vi "Program Oscillators.vi"(2 "Error In":errorcluster) -> (0 "Error Out":errorcluster)   [LabVIEW 2018]
uses:
  Type Defs/State Machine.ctl
  Type Defs/RT Command.ctl
  Type Defs/Global Action.ctl
  FGVs/Global Variables.vi
  <vilib>/Utility/config.llb/Read Key (U32).vi
  <vilib>/Utility/config.llb/Write Key (Double).vi
  <vilib>/Utility/config.llb/Write Key (Boolean).vi
  <vilib>/Utility/config.llb/NI_LVConfig.lvlib
panel:
  out "Register 0, 1, 6, 7":u32
  out "Frequncy Tuning Word":u32
  out "Register 7":u8 format="%x"
  out "Register 6":u8 format="%x"
  out "Register 5":u8 format="%x"
  out "Register 4":u8 format="%x"
  out "Register 3":u8 format="%x"
  out "Register 2":u8 format="%x"
  out "Register 1":u8 format="%x"
  out "Register 0":u8 format="%x"
  in  "Amplitude Scale Factor":dbl
  in  "Frequency Out":dbl
  in  "Reference Clock Multiplier":dbl
  in  "Reference Clock (Mhz)":dbl
  in  "DDS Select":u32(ring) items=["MP 1 - FREQ", "Q1 - FERQ", "Q2 - FREQ"]
  in  "Program Osc":bool
  in  "Current  Osc Settings":bool
  # "(160 + the Reference Clock Multipler value)"
  # "(193, the value to select single tone mode, \nDPD pin for shutdown, no SLEEP mode)"
  # "(the 1st 8 bits of the frequency tuning word)"
  # "(the 2nd 8 bits of the frequency tuning word)"
  # "(the 3rd 8 bits of the frequency tuning word)"
  # "(the last 8 bits of the frequency tuning word)"
  # "(5, the value to bypass the CIC filter)"
  # "(128 * the Amplitude Scale Factor)"
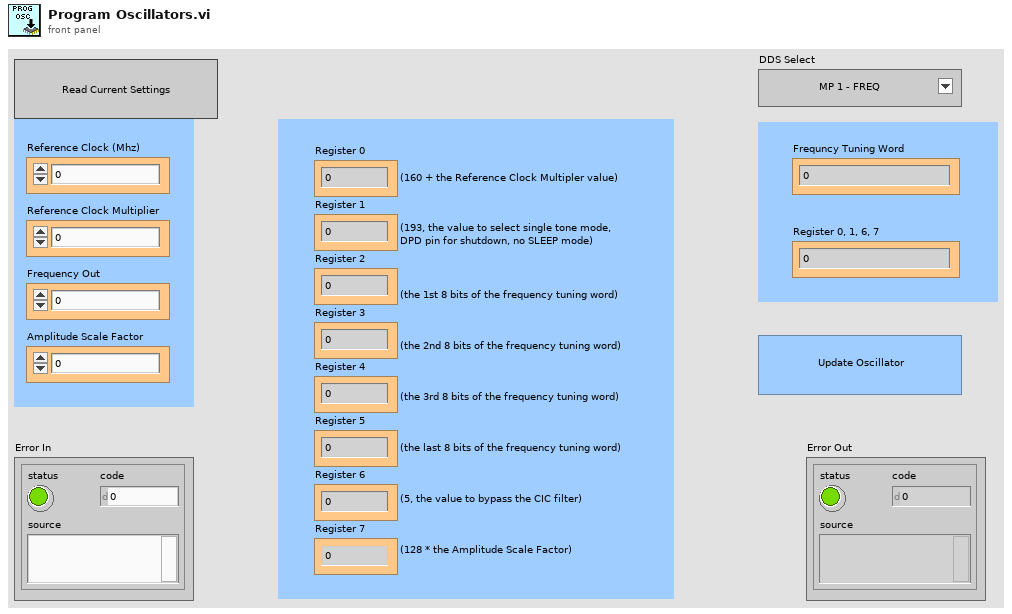
[diagram p1: front panel]
types:
  T1 = typedef "State Machine.ctl" = enum16{"Case 0", "Case 1", "Case 2", "Case 3", "Case 4", "Case 5", "Case 6", "Case 7", "Case 8", "Case 9", "Case 10", "Error", "Exit"}
  T2 = enum8{"Enabled", "Disabled", "Disabled and Grayed Out"}
  T3 = typedef "Global Action.ctl" = enum16{"Write", "Read"}
  T4 = typedef "RT Command.ctl" = enum16{"xml Start Run", "xml Start Actual Run", "xml Stop Run", "xml Runtime Update", "xml Get Status", "xml Get Table", "xml Set Table", "xml Get Configuration", "xml System Status", "xml Set LC Input Logic", "xml Get Data", "xml Get Info", "Start", "StartActualRun", "Stop", "Runtime Update", "Get Data", "Get Info", "Get Status", "Get Param", "Get Config", "Get Table", "Read ADC", "Set Oscillator", "Update Config", "Update Table", "Set All Pol", "Set Pol and DC", "Set Max Mass", "Toggle RP", "Toggle EL", "Set PIC", "Initialize Turbo", "Send Turbo Comm", "Close Turbo", "P1", "P2", "P3", "Send Serial", "Set LC Out", "Get LC In", "Read VAC", "Test Table", "Toggle Power", "Get Startup", "Set Startup", "Get ADC Table", "Set ADC Table", "Get Brief Status", "Get Detail Status", "Auxiliary Update", "Set CC Logics", "Set CC Input Logics", "Ignore Error", "invalid"}
  T5 = typedef "NI_LVConfig.lvlib/Config Data RefNum.ctl" = refnum<k1>
  T6 = typedef "Global Configrations.ctl" = cluster{"Model Name":enum16{"QSight 110", "QSight 120", "QSight 210", "QSight 220", "QSight 410", "QSight 420", "IONICS 3Q 110", "IONICS 3Q 120", "IONICS 3Q 210", "IONICS 3Q 220", "IONICS 3Q 310", "IONICS 3Q 320", "Simulation (Single Source)", "Simulation (Dual Source)"}, "RunType":u16, "Acquisition State":enum16{"Ready", "Busy", "Waiting"}, "InstrState":enum16{"Initializing", "Mass Spectrometer is Off", "Starting Up", "Turning Power Off", "Going to Standby", "Roughing Pump Ready", "Turning Turbo Off", "Turbo Startup", "Turbopump Ready", "Checking Vacuum", "Going to Ready", "Ready", "Running", "Source Standby", "Lost Communication", "Shutting Down", "Fault", "24V Standby", "Go to 24V Standby", "Turbopump Ready-Waiting"}, "Run Mode":enum16{"MRM (Q1/Q2)", "Q1 Scan", "Q1 SRM", "Q2 Scan", "Q2 SRM", "Product Scan", "Precursor Scan", "Neutral Loss", "Neutral Gain"}, "Configration":T7, "TCP ID":refnum<k5>, "DT":bool, "Dead Time (nS)":i32, "Single Source":bool, "ADC Tables":T9[]}
  T7 = typedef "Configration.ctl" = cluster{"Table":T8[], "Instrument":string[]}
  T8 = typedef "_RT Configuration 2.ctl" = cluster{"Name":string, "Ch#":u8, "Min":dbl, "Max":dbl, "Def+":dbl, "Def-":dbl, "Offset":dbl, "Slope":dbl, "Type":u8, "Description":string, "SettleT":dbl}
  T9 = typedef "ADC Table.ctl" = cluster{"Name":string, "Ch#":u8, "Min":dbl, "Max":dbl, "Def+":dbl, "Def-":dbl, "Offset":dbl, "Slope":dbl, "Type":u8, "Description":string, "SettleT":dbl}
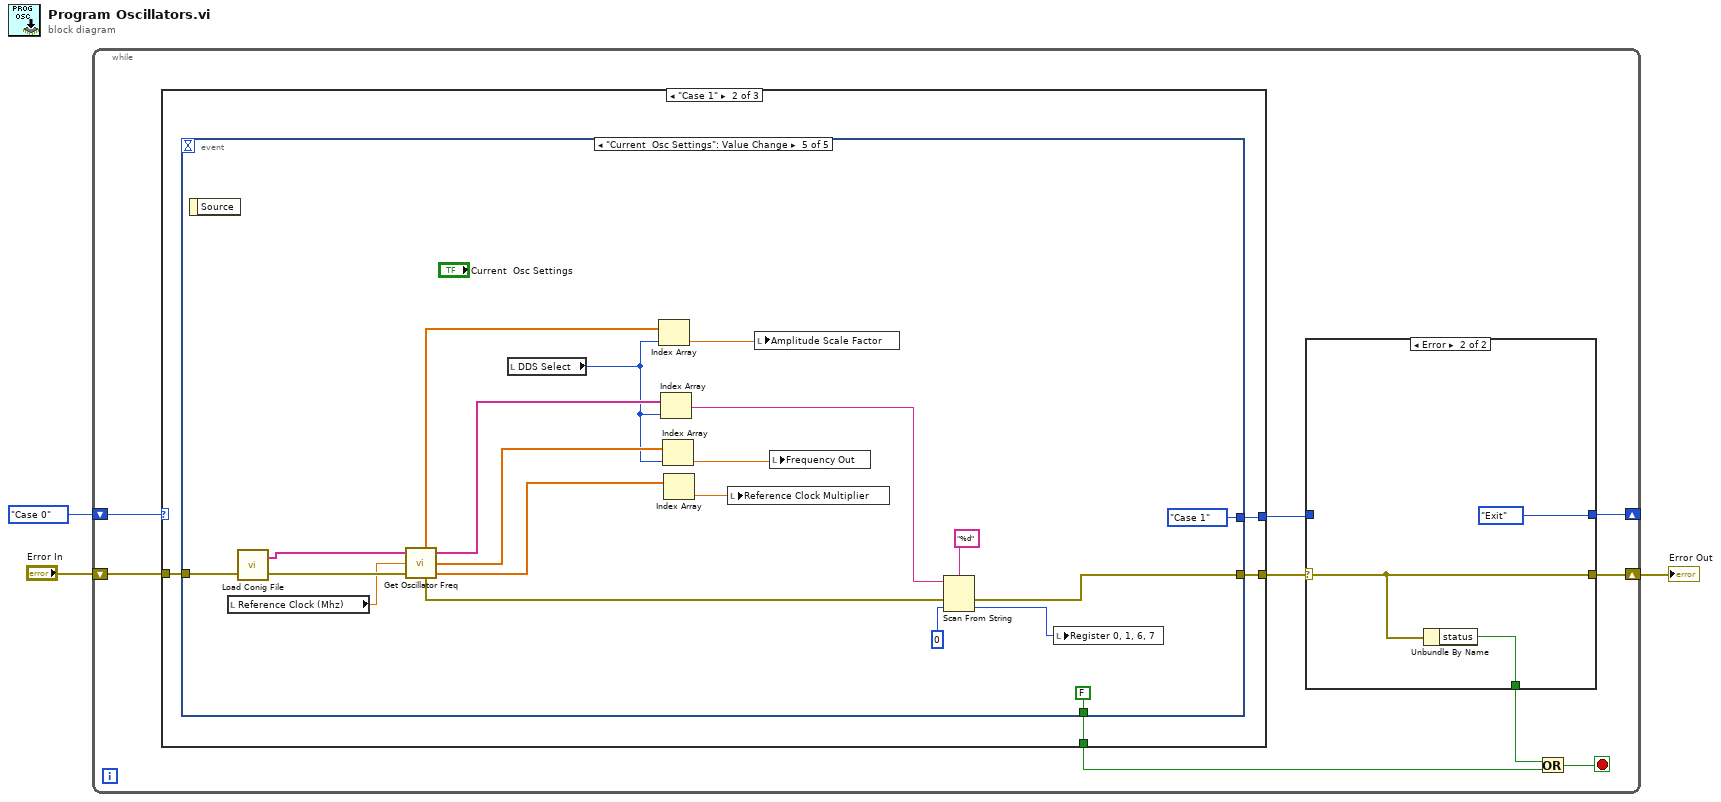
[diagram p0: block diagram]
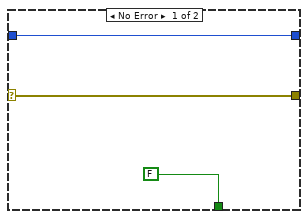
[diagram p2: hidden frame]
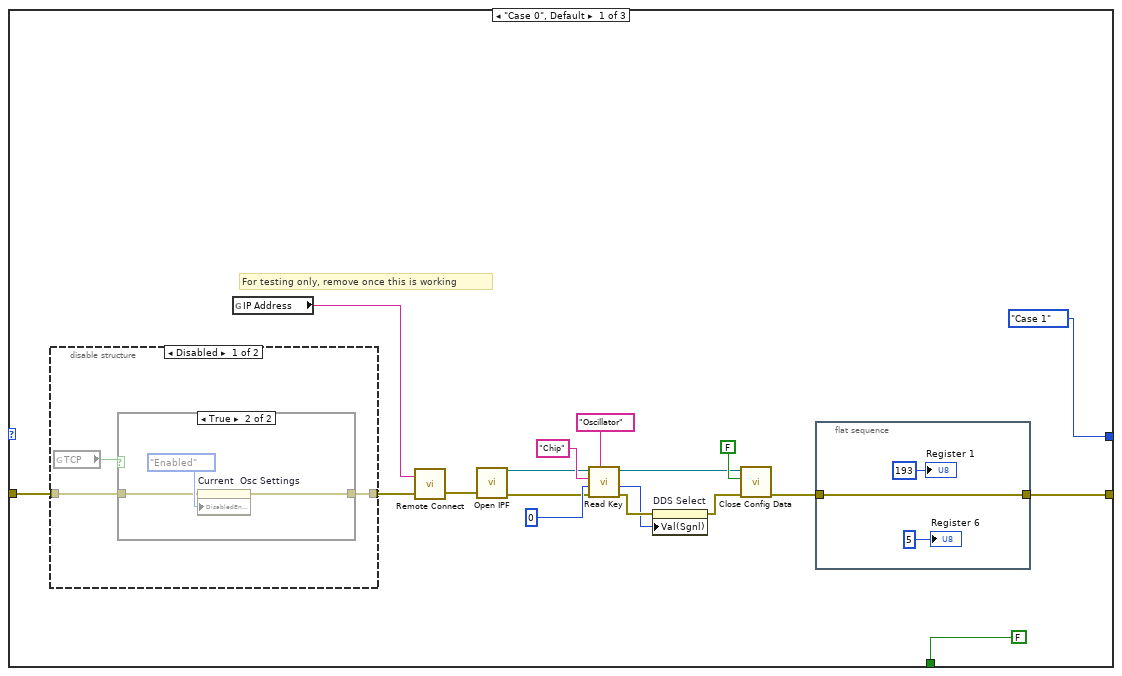
[diagram p3: hidden frame]
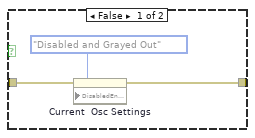
[diagram p4: hidden frame]
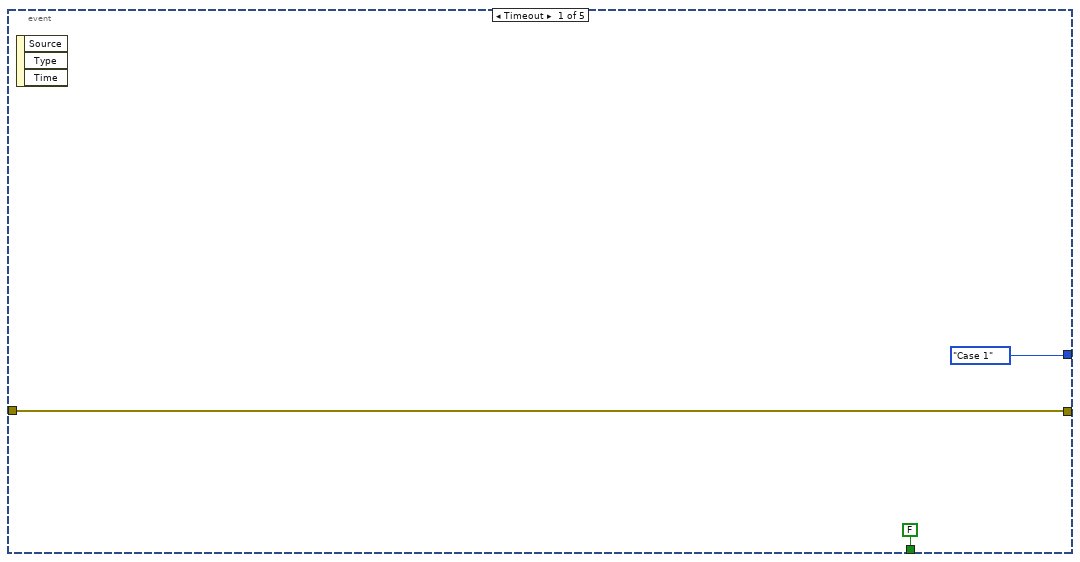
[diagram p6: hidden frame]
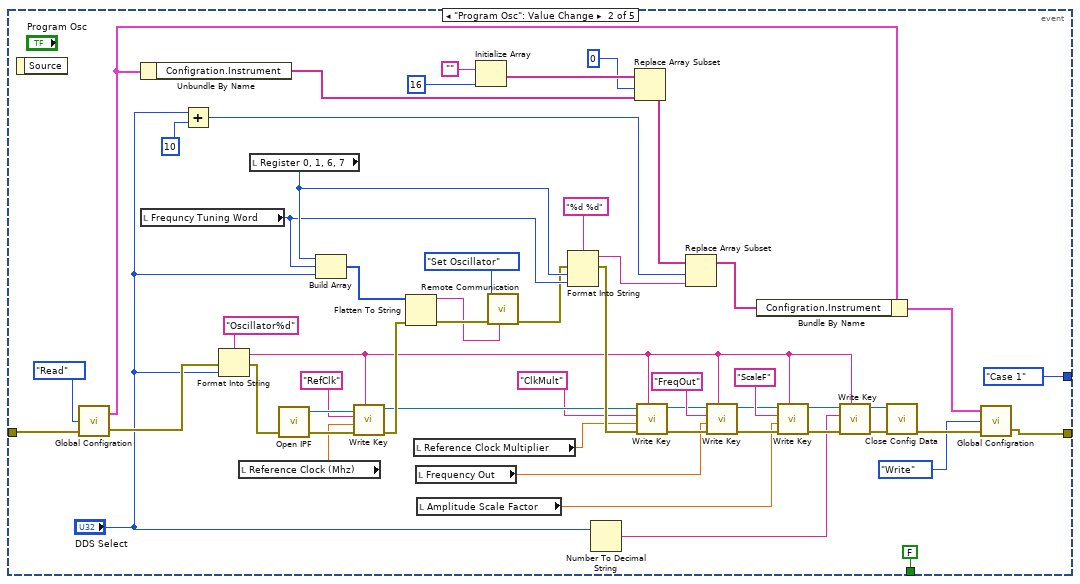
[diagram p7: hidden frame]
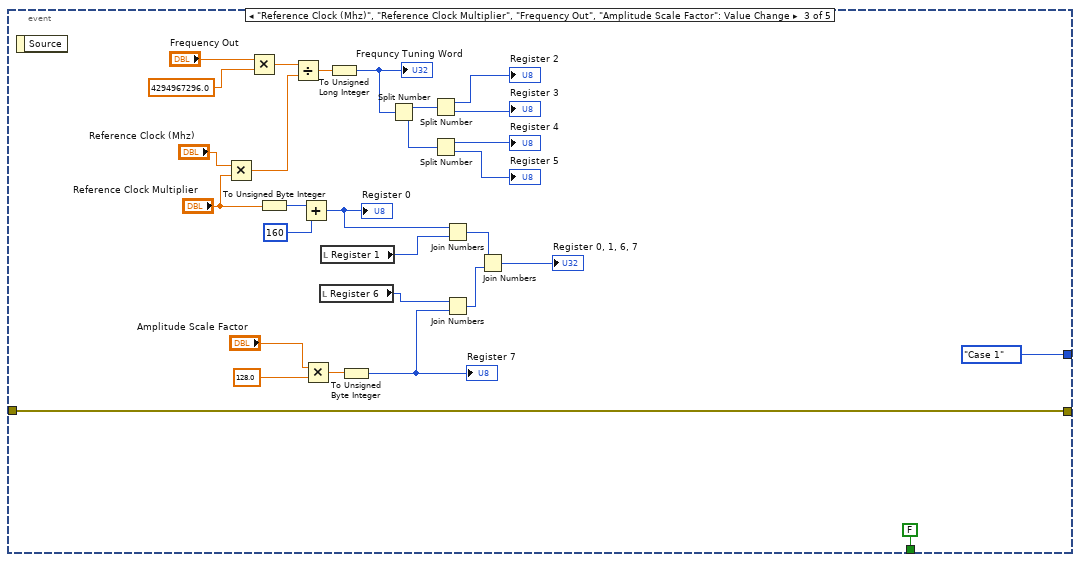
[diagram p8: hidden frame]
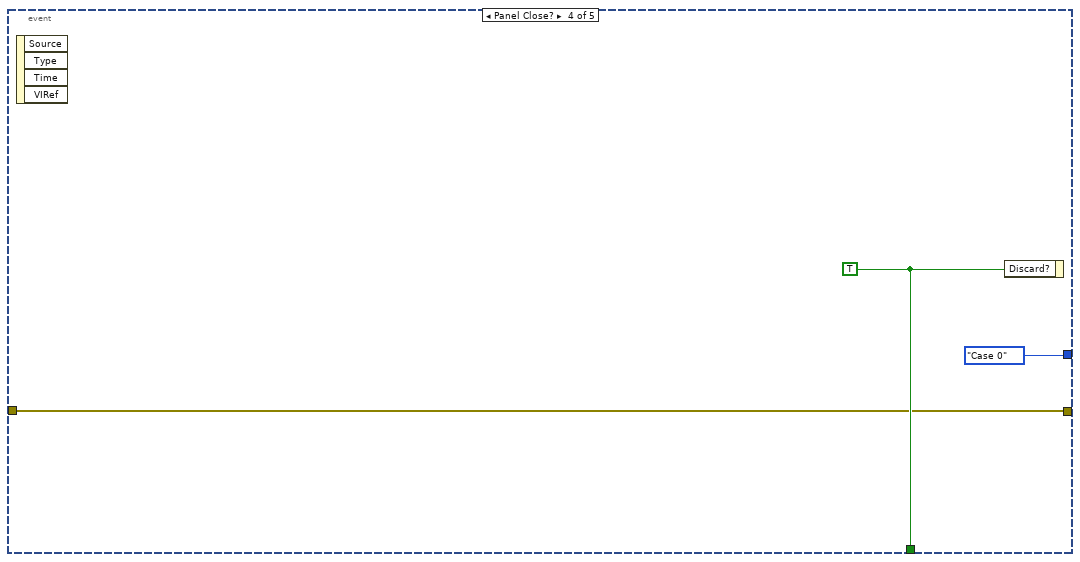
[diagram p9: hidden frame]
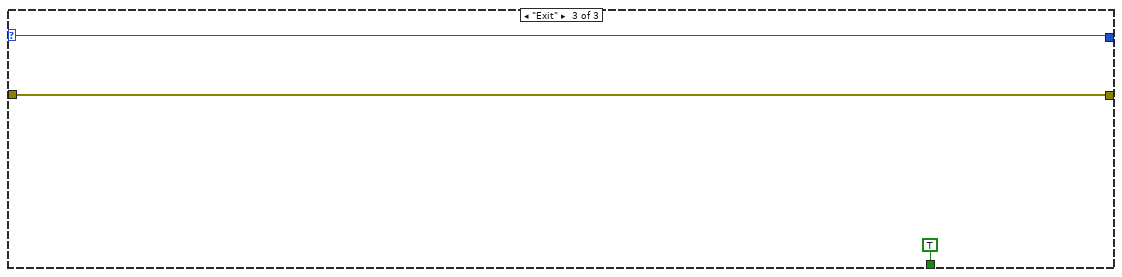
[diagram p10: hidden frame]
diagram:
  n1 = while {
    shift-right: [w9] -> w1
    shift-left: "Error In" -> [w11]
    shift-right: [w8] -> _
    shift-left: State_Machine."Case 0" ("Enum") -> [w12]
    stop <- w6 stop-if-true
    n2 = case shown="\"Case 1\"" w12 {
      selector: w12 -> [_ _ w163]
      tunnel: w11 -> [w36 w53 w164]
      tunnel: [w24 w52 w164] -> w10
      tunnel: [State_Machine."Case 1" ("Enum") w50 w163] -> w7
      tunnel: [FALSE w51 TRUE] -> w4
      frame "Case 0", Default {
        # "For testing only, remove once this is working"
        n3 = disable-structure shown="Disabled" {
          disable-tunnel: w36 -> [w38 w46]
          disable-tunnel: [w37 w46] -> w20
          frame Disabled {
            n4 = global read "Global Variables.vi" "TCP"() -> (w39:bool)
            n5 = case shown="True" w39 {
              tunnel: w38 -> [w41 w43]
              tunnel: [w40 w44] -> w37
              frame False {
                n6 = property on="Current  Osc Settings" class="Bool"(error in=w41, "DisabledEnum"=T2."Disabled and Grayed Out" ("Disabled")) -> (error out=w40:errorcluster)  [unwired: 1 in, 1 out]
              }
              frame True {
                n7 = property on="Current  Osc Settings" class="Bool"(error in=w43, "DisabledEnum"=T2."Enabled" ("Disabled")) -> (error out=w44:errorcluster)  [unwired: 1 in, 1 out]
              }
            }
          }
          frame Enabled {
          }
        }
        n8 = global read "Global Variables.vi" "IP Address"() -> (w19:string)
        n9 = call "Remote Connect.vi"("Error In"=w20, "IP Address"=w19) -> ("Error Out"=w21:errorcluster)  [unwired: 1 out]
        n10 = call "Open IPF.vi"("Error In"=w21) -> ("Error Out"=w30:errorcluster, "IPF refnum"=w23:T5)  [unwired: 2 in, 1 out]
        n11 = call-poly <vilib>:"Read Key.vi"("section"="Oscillator", "error in (no error)"=w30, "default value"=u32 0 ("Chip Select"), "key"="Chip" ("section"), "refnum"=w23) -> ("error out"=w29:errorcluster, "value"=w27:u32, "refnum out"=w33:T5)  [unwired: 4 out]
        n12 = property on="DDS Select" class="Ring (strict)"(error in=w29, "Val(Sgnl)"=w27) -> (error out=w28:errorcluster)  [unwired: 1 in, 1 out]
        n13 = call <vilib>:"Close Config Data.vi"("error in (no error)"=w28, "write file if changed (T)"=FALSE ("write configuration file? (T)"), "refnum"=w33) -> ("error out"=w25:errorcluster)  [unwired: 8 out]
        n14 = flat-sequence {
          tunnel: [w47] -> w24
          tunnel: w25 -> [w47]
          frame #0 {
            "Register 6" <- u8 5 ("Register 6")
            "Register 1" <- u8 193 ("Register 1")
          }
        }
      }
      frame "Case 1" {
        n15 = event shown="[4] \"Current  Osc Settings\": Value Change" {
          selector: _ -> [_ _ _ _ _]
          dyn-events: _ -> [_ _ _ _ _]
          timeout: _ -> [_ _ _ _ _]
          tunnel: w53 -> [w56 w79 w139 w140 w162]
          tunnel: [w56 w62 w139 w140 w151] -> w52
          tunnel: [FALSE FALSE FALSE w142 FALSE] -> w51
          tunnel: [State_Machine."Case 1" ("Enum") State_Machine."Case 1" ("Enum") State_Machine."Case 1" ("Enum") State_Machine."Case 0" ("Enum") State_Machine."Case 1" ("Enum")] -> w50
          event Timeout {
            n16 = event-data() -> ()  [unwired: 1 in, 3 out]
          }
          event "Program Osc": Value Change {
            n17 = event-data() -> ()  [unwired: 1 in, 1 out]
            n18 = call "Global Configration.vi"("Error In"=w79, "Action"=Global_Action."Read") -> ("Error Out"=w77:errorcluster, "Parameters Out"=w65:T6)  [unwired: 1 in]
            n19 = Unbundle By Name(w65) -> ("Configration.Instrument"=w68:string[])
            n20 = local read "Frequncy Tuning Word"() -> (w98:u32)
            n21 = Add(x="DDS Select", y=u32 10) -> (x+y=w70:u32)
            n22 = Format Into String(format string="Oscillator%d", error in=w77, "DDS Select") -> (resulting string=w87:string, error out=w109:errorcluster)  [unwired: 1 in]
            n23 = local read "Reference Clock (Mhz)"() -> (w106:dbl)
            n24 = local read "Register 0, 1, 6, 7"() -> (w99:u32)
            n25 = call "Open IPF.vi"("Error In"=w109) -> ("Error Out"=w108:errorcluster, "IPF refnum"=w107:T5)  [unwired: 2 in, 1 out]
            n26 = Build Array(w99, w98, "DDS Select") -> (w104:u32[])
            n27 = call-poly <vilib>:"Write Key.vi"("section"=w87, "error in (no error)"=w108, "value"=w106, "key"="RefClk" ("section"), "refnum"=w107) -> ("error out"=w103:errorcluster, "refnum out"=w94:T5)  [unwired: 3 in, 2 out]
            n28 = Flatten To String(anything=w104, error in (no error)=w103) -> (data string=w101:string, error out=w102:errorcluster)  [unwired: 3 out]
            n29 = local read "Reference Clock Multiplier"() -> (w88:dbl)
            n30 = local read "Frequency Out"() -> (w90:dbl)
            n31 = local read "Amplitude Scale Factor"() -> (w89:dbl)
            n32 = Initialize Array("", 16 ("dimension size")) -> (w72:string[])
            n33 = call "Remote Communication.vi"("String"=w101, "Error In"=w102, "Command"=RT_Command."Set Oscillator") -> ("Error Out"=w97:errorcluster)  [unwired: 3 in, 3 out]
            n34 = Format Into String(format string="%d %d", error in=w97, w99, w98) -> (resulting string=w69:string, error out=w95:errorcluster)  [unwired: 1 in]
            n35 = Number To Decimal String(number="DDS Select") -> (decimal integer string=w83:string)  [unwired: 1 out]
            n36 = Replace Array Subset(array=w72, new element=w68, index=0) -> (w71:string[])
            n37 = call-poly <vilib>:"Write Key.vi"("section"=w87, "error in (no error)"=w95, "value"=w88, "key"="ClkMult" ("section"), "refnum"=w94) -> ("error out"=w93:errorcluster, "refnum out"=w60:T5)  [unwired: 3 in, 2 out]
            n38 = Replace Array Subset(array=w71, new element=w69, index=w70) -> (w66:string[])
            n39 = call-poly <vilib>:"Write Key.vi"("section"=w87, "error in (no error)"=w93, "value"=w90, "key"="FreqOut" ("section"), "refnum"=w60) -> ("error out"=w92:errorcluster, "refnum out"=w59:T5)  [unwired: 3 in, 2 out]
            n40 = Bundle By Name(cluster=w65, "Configration.Instrument"=w66) -> (w64:T6)
            n41 = call-poly <vilib>:"Write Key.vi"("section"=w87, "error in (no error)"=w92, "value"=w89, "key"="ScaleF" ("section"), "refnum"=w59) -> ("error out"=w91:errorcluster, "refnum out"=w58:T5)  [unwired: 3 in, 2 out]
            n42 = call-poly <vilib>:"Write Key.vi"("section"=w87, "error in (no error)"=w91, "key"=w83, "refnum"=w58) -> ("error out"=w82:errorcluster, "refnum out"=w81:T5)  [unwired: 2 in, 4 out]
            n43 = call <vilib>:"Close Config Data.vi"("error in (no error)"=w82, "refnum"=w81) -> ("error out"=w80:errorcluster)  [unwired: 8 in, 1 out]
            n44 = call "Global Configration.vi"("Error In"=w80, "Action"=Global_Action."Write", "Parameters In"=w64) -> ("Error Out"=w62:errorcluster)  [unwired: 1 out]
          }
          event "Reference Clock (Mhz)", "Reference Clock Multiplier", "Frequency Out", "Amplitude Scale Factor": Value Change {
            n45 = event-data() -> ()  [unwired: 1 in, 1 out]
            n46 = Multiply(x="Reference Clock (Mhz)", y="Reference Clock Multiplier") -> (x*y=w126:dbl)
            n47 = Multiply(x="Frequency Out", y=4294967296.0) -> (x*y=w137:dbl)
            n48 = To Unsigned Byte Integer(number="Reference Clock Multiplier") -> (unsigned 8bit integer=w124:u8)
            n49 = Divide(x=w137, y=w126) -> (x/y=w136:dbl)
            n50 = Add(x=w124, y=u8 160) -> (x+y=w119:u8)
            "Register 0" <- w119
            n51 = Multiply(x="Amplitude Scale Factor", y=128.0) -> (x*y=w116:dbl)
            n52 = local read "Register 6"() -> (w118:u8)
            n53 = local read "Register 1"() -> (w120:u8)
            n54 = To Unsigned Long Integer(number=w136) -> (unsigned 32bit integer=w132:u32)
            "Frequncy Tuning Word" <- w132
            n55 = To Unsigned Byte Integer(number=w116) -> (unsigned 8bit integer=w113:u8)
            "Register 7" <- w113
            n56 = Split Number(x=w132) -> (hi(x)=w134:u16, lo(x)=w133:u16)
            n57 = Split Number(x=w134) -> (hi(x)=→"Register 2":u8, lo(x)=→"Register 3":u8)
            n58 = Split Number(x=w133) -> (hi(x)=→"Register 4":u8, lo(x)=→"Register 5":u8)
            n59 = Join Numbers(hi=w119, lo=w120) -> ((hi.lo)=w122:u16)
            n60 = Join Numbers(hi=w118, lo=w113) -> ((hi.lo)=w121:u16)
            n61 = Join Numbers(hi=w122, lo=w121) -> ((hi.lo)=→"Register 0, 1, 6, 7":u32)
          }
          event Panel Close? {
            w142 = TRUE
            n62 = event-data() -> ()  [unwired: 1 in, 4 out]
            n63 = event-data("Discard?"=w142) -> ()  [unwired: 1 in, 1 out]
          }
          event "Current  Osc Settings": Value Change {
            n64 = event-data() -> ()  [unwired: 1 in, 1 out]
            n65 = local read "Reference Clock (Mhz)"() -> (w156:dbl)
            n66 = call "Load Conig File.vi"("error in (no error)"=w162) -> ("error out"=w161:errorcluster, "Instrument"=w160:string[])  [unwired: 1 in]
            n67 = call "Get Oscillator Freq.vi"("error in (no error)"=w161, "Reference Clock"=w156, "Array 3"=w160) -> ("Reference Clock Multiplier"=w148:dbl[], "error out"=w147:errorcluster, "Oscillator Freqs"=w153:dbl[], "Tuning Word"=w155:string[], "Scaling Factor"=w154:dbl[])
            n68 = local read "DDS Select"() -> (w152:u32)
            n69 = Index Array(array=w154, index=w152) -> (element=w144:dbl)
            n70 = Index Array(array=w155, index=w152) -> (element=w159:string)
            n71 = Index Array(array=w153, index=w152) -> (element=w149:dbl)
            n72 = Index Array(array=w148) -> (element=w143:dbl)  [unwired: 1 in]
            n73 = local write "Reference Clock Multiplier"(w143) -> ()
            n74 = local write "Amplitude Scale Factor"(w144) -> ()
            n75 = local write "Frequency Out"(w149) -> ()
            n76 = Scan From String(format string="%d", input string=w159, error in=w147, default 1=u32 0 ("Frequency Tuning Word")) -> (error out=w151:errorcluster, output 1=w146:u32)  [unwired: 1 in, 2 out]
            n77 = local write "Register 0, 1, 6, 7"(w146) -> ()
          }
        }
      }
      frame "Exit" {
      }
    }
    n78 = case shown="Error" w10 {
      selector: w10 -> [w15 w17]
      tunnel: [w15 w17] -> w9
      tunnel: w7 -> [w14 _]
      tunnel: [w14 State_Machine."Exit" ("Enum")] -> w8
      tunnel: [FALSE w16] -> w5
      frame No Error {
      }
      frame Error {
        n79 = Unbundle By Name(w17) -> ("status"=w16:bool)
      }
    }
    n80 = Or(x=w5, y=w4) -> (x .or. y?=w6:bool)
  }
  "Error Out" <- w1
